vi "BW_LPF_comparison.vi"() -> ()   [LabVIEW 2022 SP3]
uses:
  <vilib>/express/express analysis/Spectral/Block/exnSpectralBlock spectral measurements peak poly.vi
  <vilib>/express/express analysis/Spectral/Block/exnSpectralBlock spectral measurements peak DDT.vi
  <vilib>/express/express analysis/Spectral/XNode/ExpressSpectralMeasurementsBlockNode.xnode
panel:
  out "Waveform":dbl[][](graph)
  out "FFT Spectrum":dbl[][](graph)
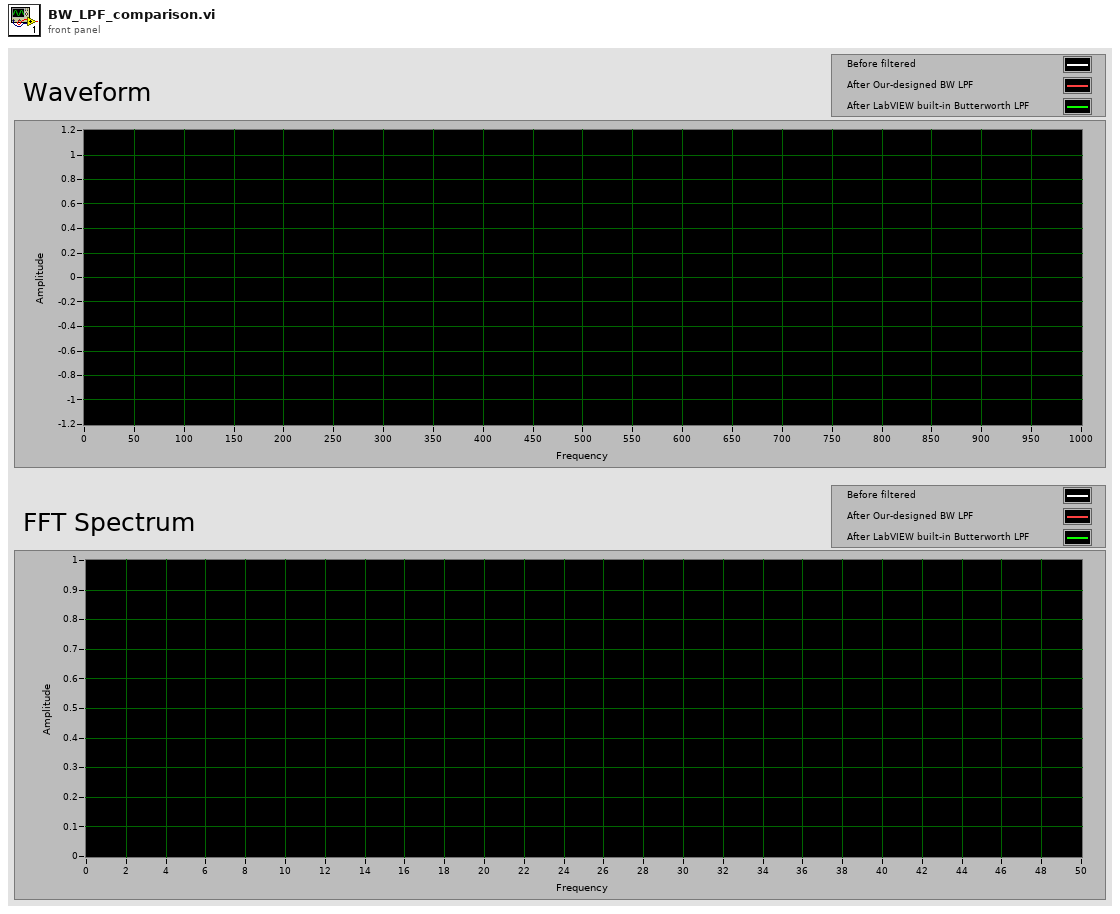
[diagram p1: front panel]
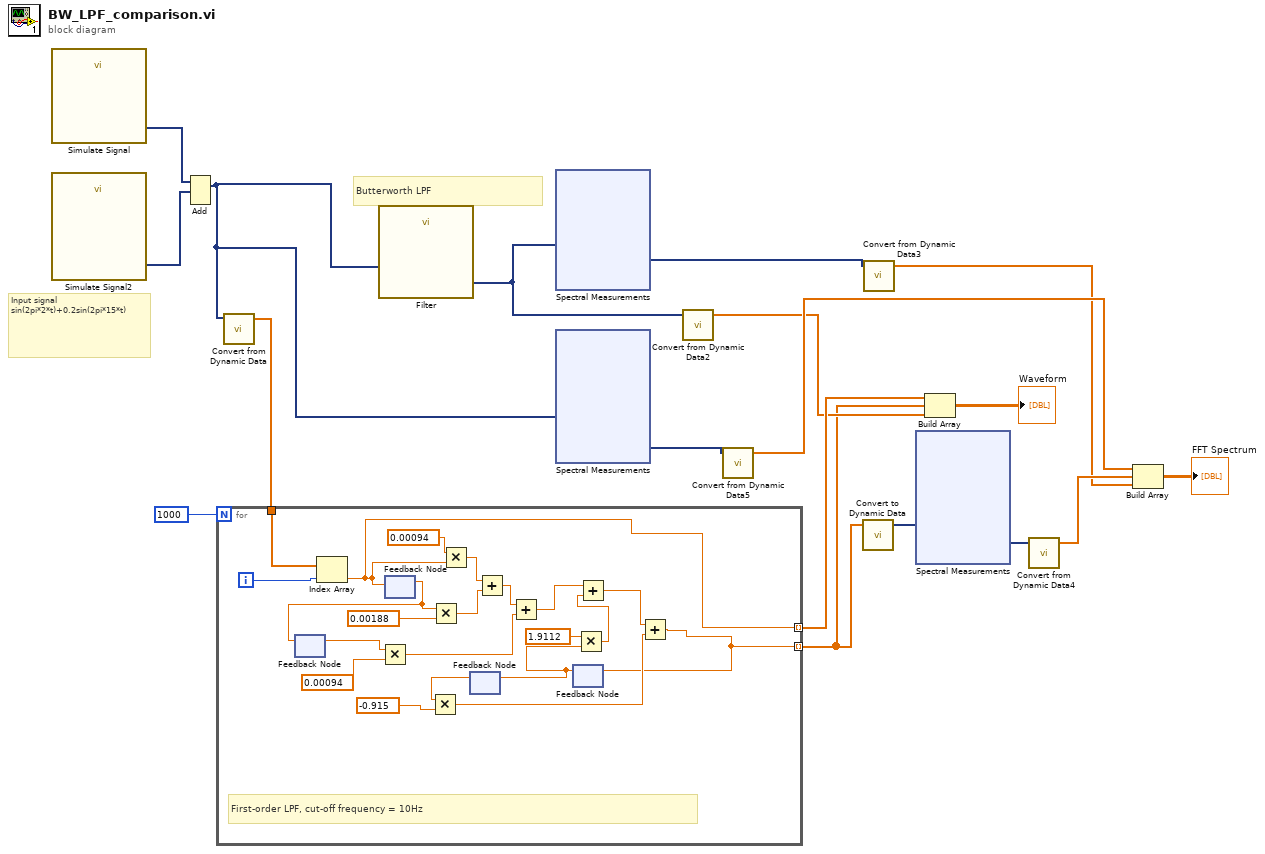
[diagram p0: block diagram]
diagram:
  # "Input signal\nsin(2pi*2*t)+0.2sin(2pi*15*t)"
  # "Butterworth LPF"
  n1 = call "Simulate Signal"() -> ("Sine"=w18:dynamicdata)  [unwired: 14 in, 1 out]
  n2 = call "Simulate Signal2"() -> ("Sine"=w17:dynamicdata)  [unwired: 14 in, 1 out]
  n3 = Add(1:w17, 2:w18) -> (0:w8:dynamicdata)  [unwired: 1 in, 1 out]
  n4 = call "Convert from Dynamic Data"("Dynamic Data Type"=w8) -> ("Array"=w15:dbl[])  [unwired: 3 in]
  n5 = for {
    N: 1000 -> [_]
    tunnel: w15 -> [w33]
    tunnel: [w31] -> w5 mode=indexing
    tunnel: [w19] -> w3 mode=indexing
    i -> [w32]
    # "First-order LPF, cut-off frequency = 10Hz"
    n6 = feedback #1() -> (w26:dbl)  [unwired: 1 in]
    n7 = Index Array(array=w33, index=w32) -> (element=w31:dbl)
    n8 = Multiply(x=w26, y=0.00094) -> (x*y=w23:dbl)
    n9 = feedback #2() -> (w27:dbl)  [unwired: 1 in]
    n10 = feedback-in #1(w27) -> ()
    n11 = feedback-in #2(w31) -> ()
    n12 = Multiply(x=w27, y=0.00188) -> (x*y=w36:dbl)
    n13 = Multiply(x=0.00094, y=w31) -> (x*y=w37:dbl)
    n14 = feedback #3() -> (w28:dbl)  [unwired: 1 in]
    n15 = Multiply(x=w28, y=-0.915) -> (x*y=w20:dbl)
    n16 = Add(x=w37, y=w36) -> (x+y=w24:dbl)
    n17 = Add(x=w24, y=w23) -> (x+y=w22:dbl)
    n18 = feedback #4() -> (w29:dbl)  [unwired: 1 in]
    n19 = feedback-in #3(w29) -> ()
    n20 = Multiply(x=1.9112, y=w29) -> (x*y=w34:dbl)
    n21 = Add(x=w22, y=w34) -> (x+y=w21:dbl)
    n22 = Add(x=w21, y=w20) -> (x+y=w19:dbl)
    n23 = feedback-in #4(w19) -> ()
  }
  n24 = call "Filter"("Signal"=w8) -> ("Filtered Signal"=w14:dynamicdata)  [unwired: 9 in, 1 out]
  n25 = xnode "Spectral Measurements"("Signals"=w14) -> ("FFT - (Peak)"=w11:dynamicdata)  [unwired: 1 in, 2 out]
  n26 = xnode "Spectral Measurements"("Signals"=w8) -> ("FFT - (Peak)"=w7:dynamicdata)  [unwired: 1 in, 2 out]
  n27 = call "Convert from Dynamic Data2"("Dynamic Data Type"=w14) -> ("Array"=w4:dbl[])  [unwired: 3 in]
  n28 = call "Convert from Dynamic Data5"("Dynamic Data Type"=w7) -> ("Array"=w6:dbl[])  [unwired: 3 in]
  n29 = call "Convert to Dynamic Data"("Array"=w3) -> ("Dynamic Data Type"=w12:dynamicdata)  [unwired: 3 in]
  n30 = call "Convert from Dynamic Data3"("Dynamic Data Type"=w11) -> ("Array"=w1:dbl[])  [unwired: 3 in]
  n31 = xnode "Spectral Measurements"("Signals"=w12) -> ("FFT - (Peak)"=w10:dynamicdata)  [unwired: 1 in, 2 out]
  n32 = Build Array(w5, w3, w4) -> (→"Waveform":dbl[][])
  n33 = call "Convert from Dynamic Data4"("Dynamic Data Type"=w10) -> ("Array"=w2:dbl[])  [unwired: 3 in]
  n34 = Build Array(w6, w2, w1) -> (→"FFT Spectrum":dbl[][])
